vi "acquire multi init subvi.vi"(8 "error in（no error）":errorcluster, 11 "VISA resource name":refnum<visa-resource-name>) -> (0 "error out":errorcluster, 1 "index":i32, 2 "read buffer":string, 3 "VISA resource name out":refnum<visa-resource-name>)   [LabVIEW 2023, in "owon.lvlib"]
uses:
  owon.lvlib
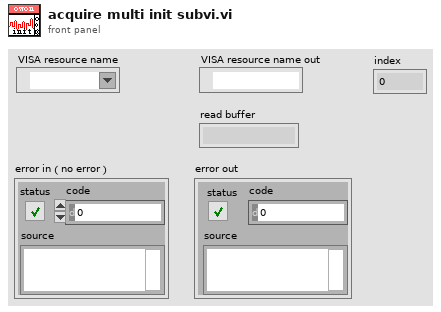
[diagram p1: front panel]
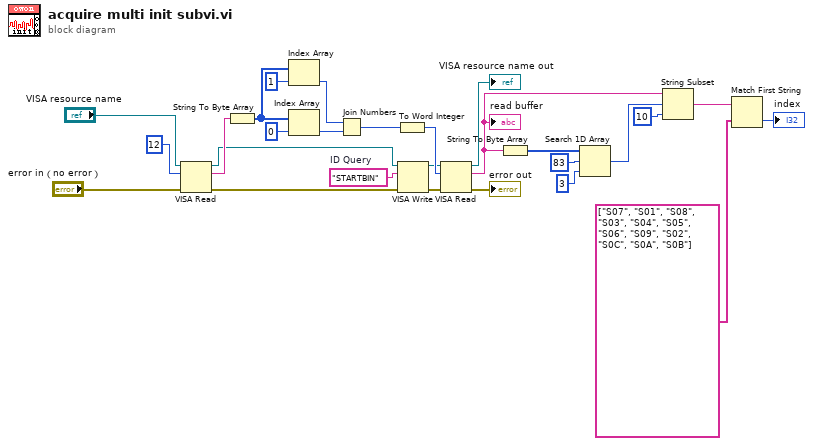
[diagram p0: block diagram]
diagram:
  w12 = "STARTBIN"  # ID Query
  n1 = VISA Read(VISA resource name="VISA resource name", byte count=u32 12, error in (no error)="error in（no error）") -> (VISA resource name out=w13:refnum<visa-resource-name>, read buffer=w20:string, error out=w14:errorcluster)  [unwired: 1 out]
  n2 = String To Byte Array(string=w20) -> (unsigned byte array=w22:u8[])
  n3 = Index Array(array=w22, index=1 ("索引")) -> (element=w24:u8)
  n4 = Index Array(array=w22, index=0 ("索引")) -> (element=w25:u8)
  n5 = Join Numbers(hi=w24, lo=w25) -> ((hi.lo)=w26:u16)
  n6 = To Word Integer(number=w26) -> (16bit integer=w27:i16)
  n7 = VISA Write(VISA resource name=w13, write buffer=w12, error in (no error)=w14) -> (VISA resource name out=w15:refnum<visa-resource-name>, error out=w16:errorcluster)  [unwired: 1 out]
  n8 = VISA Read(VISA resource name=w15, byte count=w27, error in (no error)=w16) -> (VISA resource name out=→"VISA resource name out":refnum<visa-resource-name>, read buffer=w5:string, error out=→"error out":errorcluster)  [unwired: 1 out]
  "read buffer" <- w5
  n9 = String To Byte Array(string=w5) -> (unsigned byte array=w4:u8[])
  n10 = Search 1D Array(1D array=w4, element=u8 83 ("元素"), start index (0)=3 ("开始索引(0)")) -> (index of element=w1:i32)
  n11 = String Subset(string=w5, offset (0)=w1, length (rest)=10 ("长度（剩余）")) -> (substring=w8:string)
  n12 = Match First String(2:string[] ["S07", "S01", "S08", "S03", "S04", "S05", "S06", "S09", "S02", "S0C", "S0A", "S0B"], 3:w8) -> (0:→"index":i32)  [unwired: 1 out]
